vi "Test Sever.vi"   [LabVIEW 2024]
uses:
  <vilib>/ActorFramework/Actor/Actor.lvclass
  Serve/Serve/Serve.lvclass
  C:/Program Files (x86)/National Instruments/LabVIEW 2024/vi.lib/ActorFramework/Actor/Actor.lvclass
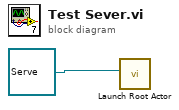
[diagram p0: block diagram]
diagram:
  n1 = call <vilib>:"Launch Root Actor.vi"("Actor"=refnum<class "Serve.lvclass"> refnum ("Serve.lvlib:Serve.lvclass")) -> ()  [unwired: 9 in, 2 out]
